vi "Begin.vi"(8 "error in":errorcluster) -> (0 "error out":errorcluster)   [LabVIEW 2015]
doc: "Called before other user functions, this VI is expected to open initial I/O refnums, load in file data, and do all program initialization. Notice that the <B>error out</B> terminal is simply used for data flow. Wiring it to other structures or subVIs ensures that this VI runs first."
uses:
  <vilib>/Rock Robotics/WPI/DriverStation/WPI_DriverStationRobotMode2.ctl
  <vilib>/Rock Robotics/SystemInterfaces/spilib/spi_bus.ctl
  <vilib>/Rock Robotics/WPI/CAN/TalonSRX/WPI_CANTalonSRX_APIControlMode.ctl
  <vilib>/Rock Robotics/SystemInterfaces/DIO/FPGA_DIOChannel.ctl
  <vilib>/Rock Robotics/WPI/CAN/TalonSRX/WPI_CANTalonSRX_APIFeedbackSelect.ctl
  <vilib>/Rock Robotics/WPI/CAN/TalonSRX/WPI_CANTalonSRX_BrakeOverride.ctl
  <vilib>/Rock Robotics/WPI/Joystick/WPI_JoystickDeviceEnum.ctl
  <vilib>/Rock Robotics/WPI/CAN/TalonSRX/WPI_CANTalonSRX_Params.ctl
  Robot Global Data.vi
  Team900-VIs/navX Library v2/IO/Open/Z900_navX_Open_SPI.vi
  <vilib>/Rock Robotics/WPI/MotorControl/WPI_MotorControlOpenCANTalonSRX.vi
  Team900-VIs/navX Library v2/navX Library v2.lvlib
panel:
  in  "Turret PID (position) Long Distance Seek":T1={"P"=0.21, "I"=0.0002, "D"=3.0, "F"=0.0, "I Zone"=1400.0}
  in  "Turret PID (position) Short distance seek":T1={"P"=0.001, "I"=0.0035, "D"=0.0, "F"=0.0, "I Zone"=1200.0}
  in  "Max Percent Throttle Turret":dbl=0.2
  in  "Speed PID":T2={"P"=0.04995, "I"=4.995e-05, "D"=0.4995, "F Left"=0.5, "F Right"=0.5}
  in  "Shooter PID Speed":T1={"P"=10.625, "I"=0.002125, "D"=0.00010625, "F"=3.81802, "I Zone"=24.0}
  in  "Revolutions per turret revolution":dbl=15.0
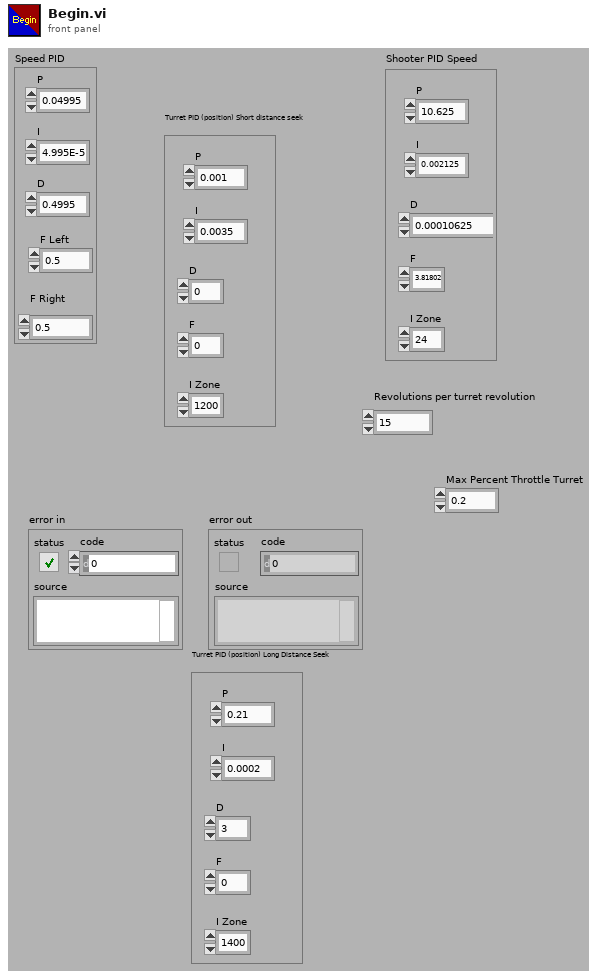
[diagram p1: front panel]
types:
  T1 = cluster{"P":dbl, "I":dbl, "D":dbl, "F":dbl, "I Zone":dbl}
  T2 = cluster{"P":dbl, "I":dbl, "D":dbl, "F Left":dbl, "F Right":dbl}
  T3 = typedef "FPGA_DIOChannel.ctl" = enum8{"DIO 0", "DIO 1", "DIO 2", "DIO 3", "DIO 4", "DIO 5", "DIO 6", "DIO 7", "DIO 8", "DIO 9", "DIO MXP 0", "DIO MXP 1", "DIO MXP 2", "DIO MXP 3", "DIO MXP 4", "DIO MXP 5", "DIO MXP 6", "DIO MXP 7", "DIO MXP 8", "DIO MXP 9", "DIO MXP 10", "DIO MXP 11", "DIO MXP 12", "DIO MXP 13", "DIO MXP 14", "DIO MXP 15", "Invalid"}
  T4 = typedef "WPI_CANTalonSRX_APIFeedbackSelect.ctl" = enum16{"Digital Quadrature Encoder", "Analog Potentiometer", "Analog Encoder", "Count on Quad-A (Rising-Edge)", "Count on Quad-A (Falling-Edge)", "CTR Magnetic Enc (Absolute)", "CTR Magnetic Enc (Relative)", "Pulse Width"}
  T5 = typedef "WPI_JoystickDeviceEnum.ctl" = enum16{"USB 0", "USB 1", "USB 2", "USB 3", "USB 4", "USB 5"}
  T6 = typedef "WPI_CANTalonSRX_BrakeOverride.ctl" = enum8{"No Override", "Override to Coast", "Override to Brake"}
  T7 = typedef "WPI_CANTalonSRX_APIControlMode.ctl" = enum8{"Percent VBus", "Speed", "Position", "Slave", "Unchanged / Invalid", "Voltage Compensation", "Current", "Motion Profile"}
  T8 = typedef "spi_bus.ctl" = enum16{"SPI On-Board, CS0", "SPI On-Board, CS1", "SPI On-Board, CS2", "SPI On-Board, CS3", "SPI MXP", "Invalid"}
  T9 = typedef "WPI_DriverStationRobotMode2.ctl" = enum16{"Autonomous Disabled", "Autonomous Enabled", "Teleop Disabled", "Teleop Enabled", "Disconnected", "Finish", "Test Disabled", "Test Enabled", "Emergency Stopped"}
  T10 = typedef "WPI_MotorControlDeviceRef.ctl" = cluster{"DeviceStatus":errorcluster, "Type":T11, "PWM":cluster{"PWM Channel":T12, "DeadBand":T13}, "CAN":cluster{"Device Number":u8, "Control Mode":T14, "Semaphore":T15, "Max Vout":dbl, "TalonSRX Control Mode":T7}, "Invert":bool}
  T11 = typedef "WPI_MotorControlType.ctl" = enum16{"PWM", "CAN", "CANTalonSRX"}
  T12 = typedef "FPGA_DIOPWMChannel.ctl" = enum8{"PWM 0", "PWM 1", "PWM 2", "PWM 3", "PWM 4", "PWM 5", "PWM 6", "PWM 7", "PWM 8", "PWM 9", "PWM MXP 0", "PWM MXP 1", "PWM MXP 2", "PWM MXP 3", "PWM MXP 4", "PWM MXP 5", "PWM MXP 6", "PWM MXP 7", "PWM MXP 8", "PWM MXP 9", "Invalid"}
  T13 = typedef "WPI_PWMDeadband.ctl" = cluster{"Name":string, "maxPositivePwm":i32, "minPositivePwm":i32, "centerPwm":i32, "maxNegativePwm":i32, "minNegativePwm":i32, "angularRange":u16}
  T14 = typedef "WPI_CANJaguar_ControlMode.ctl" = enum8{"Percent VBus", "Current", "Speed", "Position", "Voltage"}
  T15 = typedef "Semaphore RefNum" = refnum<k1>
  T16 = typedef "WPI_DigitalInputDevRef.ctl" = cluster{"DevStatus":errorcluster, "DIO Channel":T3}
  T17 = typedef "navX Library v2.lvlib/Z900_navX_DeviceTypeDef.ctl" = cluster{"Interface":cluster{"Protocol":T18, "Update Rate (4Hz-60Hz)":u8, "navX Open TypeDef":variant}, "Notify Packet":refnum<notifier>, "Loop VI Refnum":refnum<vi>, "Ready to Close Occurrence Refnum":refnum<k4>}
  T18 = typedef "navX Library v2.lvlib/Z900_navX_ProtocolTypeDef.ctl" = enum16{"SERIAL", "I2C", "SPI"}
  T19 = typedef "WPI_CANTalonSRX_Params.ctl" = u8
  T20 = typedef "WPI_JoystickDevRef.ctl" = cluster{"Device":T5}
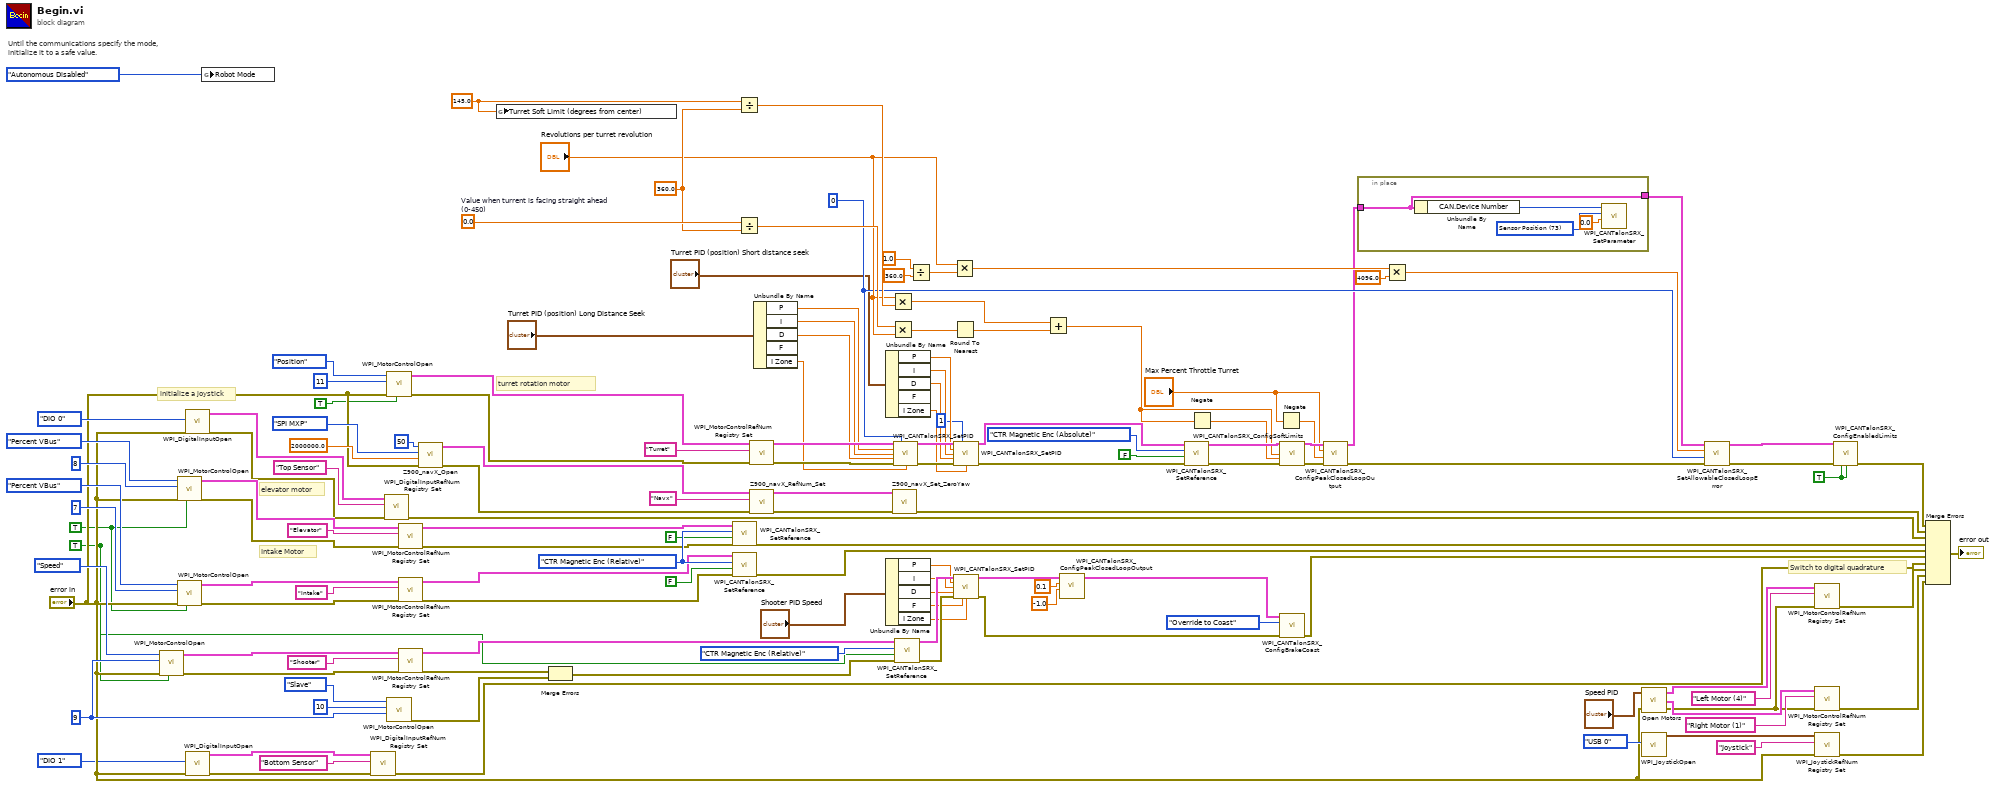
[diagram p0: block diagram]
diagram:
  w29 = 0
  w44 = 360.0 ("y")
  w47 = TRUE ("Reverse Feedback Sensor")
  w49 = TRUE ("Invert")
  w52 = TRUE
  w12 = 145.0 ("y")
  w103 = 0.0  # Value when turrent is facing straight ahead (0-450)
  w111 = u8 9 ("Master Device Number")
  w130 = WPI_CANTalonSRX_APIFeedbackSelect."CTR Magnetic Enc (Relative)" ("Feedback Reference")
  # "Switch to digital quadrature"
  # "turret rotation motor"
  # "elevator motor"
  # "Intake Motor"
  # "initialize a joystick"
  # "Until the communications specify the mode,\ninitialize it to a safe value."
  n1 = call-poly <vilib>:"WPI_MotorControlOpen.vi"("Invert"=w47, "error in (no error)"="error in", "Device Number"=w111, "Control Mode"=WPI_CANTalonSRX_APIControlMode."Speed") -> ("error out"=w101:errorcluster, "MotorControlDeviceRef"=w116:T10)  [unwired: 6 in]
  n2 = call-poly <vilib>:"WPI_MotorControlOpen.vi"("Invert"=w49, "error in (no error)"="error in", "Device Number"=8, "Control Mode"=WPI_CANTalonSRX_APIControlMode."Percent VBus") -> ("error out"=w126:errorcluster, "MotorControlDeviceRef"=w133:T10)  [unwired: 6 in]
  n3 = call-poly <vilib>:"WPI_MotorControlOpen.vi"("Invert"=w49, "error in (no error)"="error in", "Device Number"=7, "Control Mode"=WPI_CANTalonSRX_APIControlMode."Percent VBus") -> ("error out"=w123:errorcluster, "MotorControlDeviceRef"=w132:T10)  [unwired: 6 in]
  n4 = call <vilib>:"WPI_DigitalInputOpen.vi"("error in (no error)"="error in", "DIO Channel"=FPGA_DIOChannel."DIO 0") -> ("error out"=w93:errorcluster, "DigitalInputDevRef"=w119:T16)  [unwired: 8 in]
  n5 = call <vilib>:"WPI_DigitalInputOpen.vi"("error in (no error)"="error in", "DIO Channel"=FPGA_DIOChannel."DIO 1") -> ("error out"=w17:errorcluster, "DigitalInputDevRef"=w19:T16)  [unwired: 8 in]
  n6 = global write "Robot Global Data.vi" "Robot Mode"(WPI_DriverStationRobotMode2."Autonomous Disabled" ("Robot Mode")) -> ()
  n7 = call <vilib>:"WPI_DigitalInputRefNum Registry Set.vi"("error in (no error)"=w17, "refnum name"="Bottom Sensor", "DigitalInputDevRef"=w19) -> ("error out"=w87:errorcluster)  [unwired: 7 in, 1 out]
  n8 = call <vilib>:"WPI_DigitalInputRefNum Registry Set.vi"("error in (no error)"=w93, "refnum name"="Top Sensor", "DigitalInputDevRef"=w119) -> ("error out"=w92:errorcluster)  [unwired: 7 in, 1 out]
  n9 = call-poly <vilib>:"WPI_MotorControlOpen.vi"("Invert"=TRUE, "error in (no error)"="error in", "Device Number"=u8 11 ("Master Device Number"), "Control Mode"=WPI_CANTalonSRX_APIControlMode."Position") -> ("error out"=w95:errorcluster, "MotorControlDeviceRef"=w98:T10)  [unwired: 6 in]
  n10 = call-poly <vilib>:"WPI_MotorControlOpen.vi"("Master Device Number"=w111, "Device Number"=u8 10 ("Master Device Number"), "Control Mode"=WPI_CANTalonSRX_APIControlMode."Slave") -> ("error out"=w110:errorcluster)  [unwired: 7 in, 1 out]
  n11 = call <vilib>:"WPI_MotorControlRefNum Registry Set.vi"("error in (no error)"=w126, "refnum name"="Elevator", "MotorControlDevRef"=w133) -> ("error out"=w127:errorcluster, "MotorControlDevRef"=w128:T10)  [unwired: 7 in]
  n12 = call <vilib>:"WPI_MotorControlRefNum Registry Set.vi"("error in (no error)"=w123, "refnum name"="Intake", "MotorControlDevRef"=w132) -> ("error out"=w122:errorcluster, "MotorControlDevRef"=w124:T10)  [unwired: 7 in]
  n13 = call <vilib>:"WPI_MotorControlRefNum Registry Set.vi"("error in (no error)"=w101, "refnum name"="Shooter", "MotorControlDevRef"=w116) -> ("error out"=w100:errorcluster, "MotorControlDevRef"=w102:T10)  [unwired: 7 in]
  n14 = call-poly "Z900_navX_Open.vi"("error in (no error)"="error in", "Clock Rate (Hz)"=2000000.0, "SPI Bus"=spi_bus."SPI MXP", "Update Rate (4Hz-60Hz)"=u8 50) -> ("error out"=w72:errorcluster, "navX Device"=w73:T17)  [unwired: 6 in]
  n15 = global write "Robot Global Data.vi" "Turret Soft Limit (degrees from center)"(w12) -> ()
  n16 = Merge Errors(w100, w110) -> (w109:errorcluster)
  n17 = call <vilib>:"WPI_CANTalonSRX_SetReference.vi"("error in (no error)"=w127, "Reverse Feedback Sensor"=FALSE, "Feedback Reference"=w130, "CAN Talon SRX Ref"=w128) -> ("error out"=w91:errorcluster)  [unwired: 6 in, 1 out]
  n18 = call <vilib>:"WPI_CANTalonSRX_SetReference.vi"("error in (no error)"=w122, "Reverse Feedback Sensor"=FALSE, "Feedback Reference"=w130, "CAN Talon SRX Ref"=w124) -> ("error out"=w90:errorcluster)  [unwired: 6 in, 1 out]
  n19 = Divide(x=w12, y=w44) -> (x/y=w45:dbl)
  n20 = Divide(x=w103, y=w44) -> (x/y=w46:dbl)
  n21 = call <vilib>:"WPI_MotorControlRefNum Registry Set.vi"("error in (no error)"=w95, "refnum name"="Turret", "MotorControlDevRef"=w98) -> ("error out"=w94:errorcluster, "MotorControlDevRef"=w96:T10)  [unwired: 7 in]
  n22 = call "Z900_navX_RefNum_Set.vi"("error in (no error)"=w72, "refnum name"="Navx", "navX Device"=w73) -> ("error out"=w23:errorcluster, "navX Device"=w24:T17)  [unwired: 7 in]
  n23 = Unbundle By Name("Turret PID (position) Long Distance Seek") -> ("P"=w81:dbl, "I"=w80:dbl, "D"=w79:dbl, "I Zone"=w78:dbl)  [unwired: 1 out]
  n24 = Unbundle By Name("Turret PID (position) Short distance seek") -> ("P"=w5:dbl, "I"=w4:dbl, "D"=w3:dbl, "I Zone"=w2:dbl)  [unwired: 1 out]
  n25 = Unbundle By Name("Shooter PID Speed") -> ("P"=w86:dbl, "I"=w85:dbl, "D"=w84:dbl, "F"=w83:dbl, "I Zone"=w82:dbl)
  n26 = Multiply(x="Revolutions per turret revolution", y=w45) -> (x*y=w54:dbl)
  n27 = Multiply(x=w46, y="Revolutions per turret revolution") -> (x*y=w104:dbl)
  n28 = call "Z900_navX_Set_ZeroYaw.vi"("error in (no error)"=w23, "navX Device"=w24) -> ("error out"=w22:errorcluster)  [unwired: 8 in, 1 out]
  n29 = call <vilib>:"WPI_CANTalonSRX_SetPID.vi"("CAN Talon SRX Ref"=w96, "Parameter Slot"=w29, "P"=w81, "I"=w80, "D"=w79, "error in (no error)"=w94, "I Zone"=w78) -> ("CAN Talon SRX Ref"=w10:T10, "error out"=w8:errorcluster)  [unwired: 7 in]
  n30 = call <vilib>:"WPI_CANTalonSRX_SetReference.vi"("error in (no error)"=w109, "Reverse Feedback Sensor"=w47, "Feedback Reference"=WPI_CANTalonSRX_APIFeedbackSelect."CTR Magnetic Enc (Relative)", "CAN Talon SRX Ref"=w102) -> ("error out"=w108:errorcluster, "CAN Talon SRX Ref"=w106:T10)  [unwired: 6 in]
  n31 = Divide(x=1.0, y=360.0) -> (x/y=w32:dbl)
  n32 = Multiply(x="Revolutions per turret revolution", y=w32) -> (x*y=w30:dbl)
  n33 = Round To Nearest(number=w104) -> (nearest integer value=w53:dbl)
  n34 = call <vilib>:"WPI_CANTalonSRX_SetPID.vi"("CAN Talon SRX Ref"=w10, "Parameter Slot"=u8 1, "P"=w5, "I"=w4, "D"=w3, "error in (no error)"=w8, "I Zone"=w2) -> ("CAN Talon SRX Ref"=w9:T10, "error out"=w7:errorcluster)  [unwired: 7 in]
  n35 = call <vilib>:"WPI_CANTalonSRX_SetPID.vi"("CAN Talon SRX Ref"=w106, "P"=w86, "I"=w85, "D"=w84, "error in (no error)"=w108, "F"=w83, "I Zone"=w82) -> ("CAN Talon SRX Ref"=w16:T10, "error out"=w107:errorcluster)  [unwired: 7 in]
  n36 = Add(x=w54, y=w53) -> (x+y=w43:dbl)
  n37 = call <vilib>:"WPI_CANTalonSRX_ConfigPeakClosedLoopOutput.vi"("Reverse Peak Output"=-1.0, "Forward Peak Output"=0.1, "CAN Talon SRX Ref"=w16) -> ("CAN Talon SRX Ref"=w15:T10)  [unwired: 7 in, 1 out]
  n38 = call <vilib>:"WPI_CANTalonSRX_SetReference.vi"("error in (no error)"=w7, "Reverse Feedback Sensor"=FALSE, "Feedback Reference"=WPI_CANTalonSRX_APIFeedbackSelect."CTR Magnetic Enc (Absolute)", "CAN Talon SRX Ref"=w9) -> ("error out"=w57:errorcluster, "CAN Talon SRX Ref"=w58:T10)  [unwired: 6 in]
  n39 = Negate(x=w43) -> (-x=w55:dbl)
  n40 = Negate(x="Max Percent Throttle Turret") -> (-x=w41:dbl)
  n41 = call <vilib>:"WPI_CANTalonSRX_ConfigSoftLimits.vi"("CAN Talon SRX Ref"=w58, "Forward Limit Position"=w43, "Reverse Limit Position"=w55, "error in (no error)"=w57) -> ("CAN Talon SRX Ref"=w50:T10, "error out"=w40:errorcluster)  [unwired: 10 in]
  n42 = call <vilib>:"WPI_CANTalonSRX_ConfigBrakeCoast.vi"("error in (no error)"=w107, "Brake / Coast Mode"=WPI_CANTalonSRX_BrakeOverride."Override to Coast", "CAN Talon SRX Ref"=w15) -> ("error out"=w89:errorcluster)  [unwired: 7 in, 1 out]
  n43 = call <vilib>:"WPI_CANTalonSRX_ConfigPeakClosedLoopOutput.vi"("error in (no error)"=w40, "Reverse Peak Output"=w41, "Forward Peak Output"="Max Percent Throttle Turret", "CAN Talon SRX Ref"=w50) -> ("error out"=w36:errorcluster, "CAN Talon SRX Ref"=w26:T10)  [unwired: 6 in]
  n44 = in-place {
    in-place-border: w26 -> [w142]
    in-place-border: [w142] -> w25
    w140 = T19 73 items=["Slot 0 - P"=1, "Slot 0 - I"=2, "Slot 0 - D"=3, "Slot 0 - F"=4, "Slot 0 - I Zone"=5, "Slot 0 - Ramp Rate"=6, "Slot 1 - P"=11, "Slot 1 - I"=12, "Slot 1 - D"=13, "Slot 1 - F"=14, "Slot 1 - I Zone"=15, "Slot 1 - Ramp Rate"=16, "Soft Limit - Forward"=21, "Soft Limit - Reverse"=22, "On Boot - Brake Mode"=31, "On Boot - Limit Normally Closed - Forward"=32, "On Boot - Limit Normally Closed - Reverse"=33, "On Boot - Limit Disabled - Forward"=34, "On Boot - Limit Disabled - Reverse"=35, "Fault - Over Temp"=41, "Fault - Under Voltage"=42, "Fault - Forward Limit"=43, "Fault - Reverse Limit"=44, "Fault - Hardware Failure"=45, "Fault - Forward Soft Limit"=46, "Fault - Reverse Soft Limit"=47, "Sticky Fault - Over Temp"=48, "Sticky Fault - Under Voltage"=49, "Sticky Fault - Forward Limit"=50, "Sticky Fault - Reverse Limit"=51, "Sticky Fault - Forward Soft Limit"=52, "Sticky Fault - Reverse Soft Limit"=53, "Applied Throttle"=61, "Closed-Loop Error"=62, "Select Feedback Device"=63, "Reverse Closed-Loop Output"=64, "Mode Select"=65, "Profile Slot Select"=66, "Ramp Throttle"=67, "Reverse Feedback Sensor"=68, "Limit Switch Enabled"=69, "Limit Switch Closed - Forward"=70, "Limit Switch Closed - Reverse"=71, "Sensor Position"=73, "Sensor Velocity"=74, "Current"=75, "Brake is Enabled"=76, "Encoder Position"=77, "Encoder Velocity"=78, "Encoder Index Rise Events"=79, "Encoder A Pin State"=80, "Encoder B Pin State"=81, "Encoder Index Pin State"=82, "Analog In with Overflow"=83, "Analog In Velocity"=84, "Temperature"=85, "Battery Voltage"=86, "Reset Count"=87, "Reset Flags"=88, "Firmware Version"=89, "Settings Changed"=90] ("Parameter")
    n45 = Unbundle By Name(w142) -> ("CAN.Device Number"=w141:u8)
    n46 = call <vilib>:"WPI_CANTalonSRX_SetParameter.vi"("Value"=0.0, "Parameter"=w140, "Device ID (0)"=w141) -> ()  [unwired: 7 in, 2 out]
  }
  n47 = Multiply(x=w30, y=4096.0) -> (x*y=w28:dbl)
  n48 = call "Open Motors.vi"("error in"="error in", "Speed PID"="Speed PID") -> ("error out"=w67:errorcluster, "Right Motor Refs"=w68:T10, "Left Motor Refs"=w71:T10)  [unwired: 1 in]
  n49 = call <vilib>:"WPI_JoystickOpen.vi"("JoystickDevice"=WPI_JoystickDeviceEnum."USB 0") -> ("JoystickDevRef"=w63:T20)  [unwired: 10 in]
  n50 = call <vilib>:"WPI_CANTalonSRX_SetAllowableClosedLoopError.vi"("error in (no error)"=w36, "Parameter Slot"=w29, "Allowable Closed-Loop Error"=w28, "CAN Talon SRX Ref"=w25) -> ("error out"=w35:errorcluster, "CAN Talon SRX Ref"=w37:T10)  [unwired: 6 in]
  n51 = call <vilib>:"WPI_MotorControlRefNum Registry Set.vi"("error in (no error)"=w67, "refnum name"="Left Motor (4)", "MotorControlDevRef"=w71) -> ("error out"=w66:errorcluster)  [unwired: 7 in, 1 out]
  n52 = call <vilib>:"WPI_MotorControlRefNum Registry Set.vi"("error in (no error)"=w67, "refnum name"="Right Motor (1)", "MotorControlDevRef"=w68) -> ("error out"=w65:errorcluster)  [unwired: 7 in, 1 out]
  n53 = call <vilib>:"WPI_JoystickRefNum Registry Set.vi"("error in (no error)"="error in", "refnum name"="Joystick", "JoystickDevRef"=w63) -> ("error out"=w60:errorcluster)  [unwired: 7 in, 1 out]
  n54 = call <vilib>:"WPI_CANTalonSRX_ConfigEnabledLimits.vi"("CAN Talon SRX Ref"=w37, "error in (no error)"=w35, "Forward Soft Limit Enable"=w52, "Reverse Soft Limit Enable"=w52) -> ("error out"=w51:errorcluster)  [unwired: 10 in, 1 out]
  n55 = Merge Errors(w51, w22, w92, w91, w90, w89, w87, w66, w65, w60) -> (→"error out":errorcluster)
